vi "dscADSetSettings.vi"(8 "error in":errorcluster, 10 "adSettingsIn":T1, 11 "boardIn":i16) -> (0 "error out":errorcluster, 2 "adSettingsOut":T1, 3 "boardOut":i16)   [LabVIEW 2011, in "Diamond Universal Driver.lvlib"]
doc: "Set the A/D configuration for future A/D conversions. A delay of approximately 10 us occurs during this function call in order to allow the analog circuit to settle on the new settings. On -AT boards, if adsettings->load_cal == true, then load the A/D calibrations settings from the EEPROM for the current A/D range. This results in slightly more accurate A/D conversions but causes an additional, longer delay of approximately 10 ms."
uses:
  Diamond Universal Driver.lvlib
  Controls/dscADSettings.ctl
  Controls/gain.ctl
  Controls/error codes.ctl
  Instruments/WL OPC/Support/dlls/dscud.dll
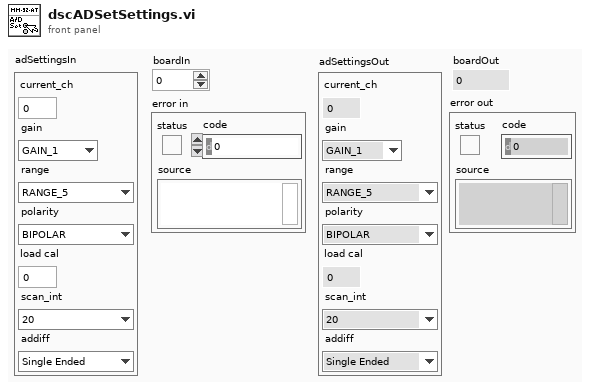
[diagram p1: front panel]
types:
  T1 = typedef "dscADSettings.ctl" = cluster{"current_ch":u8, "gain":T2, "range":enum8{"RANGE_5", "RANGE_10"}, "polarity":enum16{"BIPOLAR", "UNIPOLAR"}, "load cal":u8, "scan_int":enum8{"20", "15", "10", "5", "9", "4"}, "addiff":enum8{"Single Ended", "Differential"}}
  T2 = typedef "gain.ctl" = enum8{"GAIN_1", "GAIN_2", "GAIN_8"}
  T3 = typedef "Diamond Universal Driver.lvlib/error codes.ctl" = enum8{"DE_NONE", "DE_HW_FAILURE", "DE_SW_FAILURE", "DE_HW_NOT_SUPPORTED", "DE_SW_NOT_SUPPORTED", "DE_INVALID_PARM", "DE_ALTERNATE_IN_PROGRESS", "DE_NONE_IN_PROGRESS", "DE_BUFFER_ROLLOVER", "DE_INVALID_ERROR_CODE", "DE_ALREADY_PAUSED", "DE_OVERFLOW", "DE_INVALID_FUNC", "DE_DSCUDH_INVALID", "DE_INVALID_BOARD", "DE_BOARD_LIMIT_REACHED", "DE_BOARD_BUSY", "DE_INVALID_WINDRVR_HANDLE", "DE_INVALID_WINDRVR_VERSION", "DE_BAD_WINDRVR_BOARD_INIT", "DE_OPERATION_TIMED_OUT", "DE_INVALID_WINDRVR_KP", "DE_THREAD_FAILURE"}
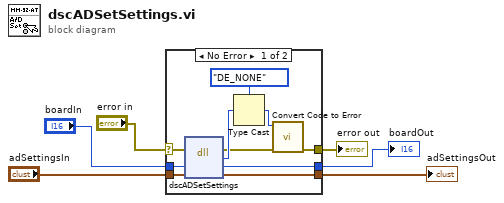
[diagram p0: block diagram]
diagram:
  n1 = case shown="No Error" "error in" {
    selector: "error in" -> [w8 w17]
    tunnel: "adSettingsIn" -> [w16 w18]
    tunnel: "boardIn" -> [w15 w19]
    tunnel: [w14 w18] -> w4
    tunnel: [w9 w17] -> w3
    tunnel: [w7 w19] -> w1
    frame No Error {
      n2 = dll-call lib="C:/Users/mrichardson/Documents/Web Based Version Control SW/Instruments/WL OPC/Support/dlls/dscud.dll" fn="dscADSetSettings"(error in=w8, "board"=w15, "adsettings"=w16) -> (error out=w10:errorcluster, "error"=w13:u8, "board"=w7:i16, "adsettings"=w14:T1)  [unwired: 2 in, 1 out]
      n3 = Type Cast(type=error_codes."DE_NONE" ("error codes"), x=w13) -> (*(type *) &x=w11:T3)
      n4 = call "Convert Code to Error.vi"("error in"=w10, "error codes"=w11) -> ("error out"=w9:errorcluster)  [unwired: 9 in]
    }
    frame Error {
    }
  }
  "adSettingsOut" <- w4
  "error out" <- w3
  "boardOut" <- w1
